vi "Thingworx_Read.vi"(11 "Thingworx":string(xcontrol)) -> (1 "number":dbl, 2 "value":string)   [LabVIEW 2019]
uses:
  _TW_Subs/TW_XControl.xctl
panel:
  out "new picture":picture
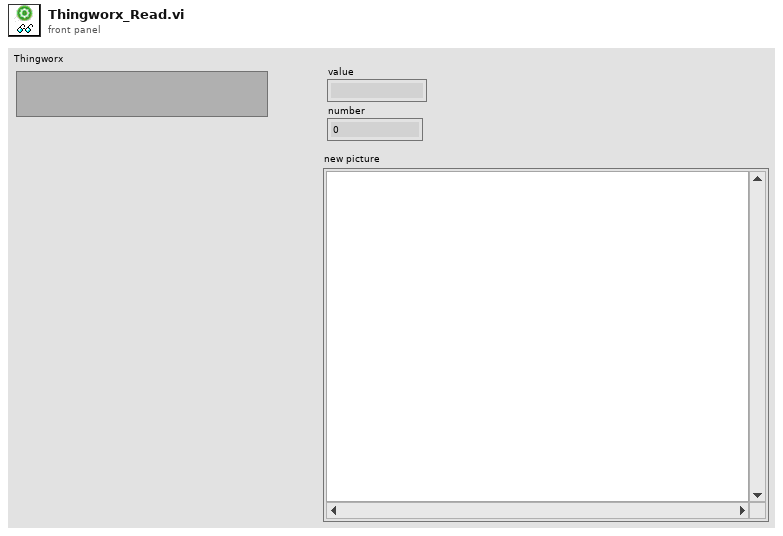
[diagram p1: front panel]
types:
  T1 = typedef "imagedata.ctl" = cluster{"image type":i32, "image depth":i32, "image":u8[], "mask":u8[], "colors":u32[], "Rectangle":cluster{"left":i16, "top":i16, "right":i16, "bottom":i16}}
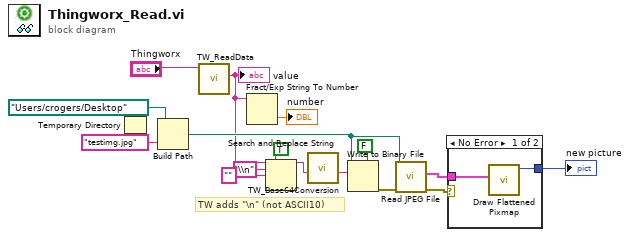
[diagram p0: block diagram]
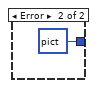
[diagram p2: hidden frame]
diagram:
  # "TW adds \"\\n\" (not ASCII10)"
  n1 = Temporary Directory() -> ()  [unwired: 1 out]
  n2 = Build Path(base path=path "/Users/crogers/Desktop", name or relative path="testimg.jpg") -> (appended path=w9:path)
  n3 = call "TW_ReadData.vi"("Property"="Thingworx") -> ("value"=w4:string)  [unwired: 10 in]
  "value" <- w4
  n4 = Fract/Exp String To Number(string=w4) -> (number=→"number":dbl)  [unwired: 3 in, 1 out]
  n5 = Search and Replace String(replace all?=TRUE ("replace all? (F)"), input string=w4, search string="\\n", replace string="" ("replace string (\"\")")) -> (result string=w3:string)  [unwired: 4 in, 3 out]
  n6 = call "TW_Base64Conversion.vi"("Base64 String in"=w3) -> ("String out"=w8:string)  [unwired: 8 in, 2 out]
  n7 = Write to Binary File(file (use dialog)=w9, data=w8, 5:FALSE ("prepend array or string size? (T)")) -> (error out=w13:errorcluster)  [unwired: 3 in, 2 out]
  n8 = call <vilib>:"Read JPEG File.vi"("error in (no error)"=w13, "path to JPEG file"=w9) -> ("error out"=w1:errorcluster, "image data"=w12:T1)  [unwired: 7 in, 1 out]
  n9 = case shown="No Error" w1 {
    tunnel: w12 -> [w18 _]
    tunnel: [w17 picture data[5B] ("new picture")] -> w11
    frame No Error {
      n10 = call <vilib>:"Draw Flattened Pixmap.vi"("image data"=w18) -> ("new picture"=w17:picture)  [unwired: 8 in]
    }
    frame Error {
    }
  }
  "new picture" <- w11
